vi "Binary Number Mantissa and Exponent (U8).vi"(7 "Binary Number":u8 format="%08b") -> (6 "Exponent (-N)":u8, 8 "Mantissa (M)":u8 format="%08b")   [LabVIEW 2010]
panel:
  out "One Hot Encoded Number":u8 format="%08b"
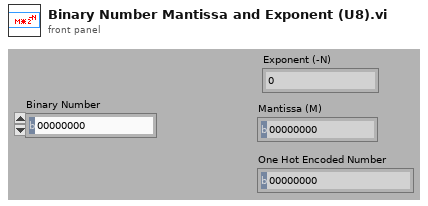
[diagram p1: front panel]
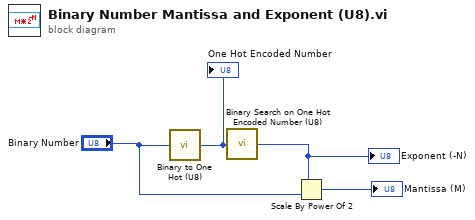
[diagram p0: block diagram]
diagram:
  n1 = call "Binary to One Hot (U8).vi"("Binary Number"="Binary Number") -> ("One Hot Encoded Number"=w4:u8)  [unwired: 14 in]
  "One Hot Encoded Number" <- w4
  n2 = call "Binary Search on One Hot Encoded Number (U8).vi"("One Hot Encoded Number"=w4) -> ("Binary Number"=w1:u8)  [unwired: 14 in]
  "Exponent (-N)" <- w1
  n3 = Scale By Power Of 2(n=w1, x="Binary Number") -> (x*2^n=→"Mantissa (M)":u8)
